vi "nn sendmsg.vi"(8 "error in (no error)":errorcluster, 9 "flags":i32, 10 "msghdr":T1, 11 "s":i32) -> (0 "error out":errorcluster, 3 "function return":i32)   [LabVIEW 2013, in "lvnano.lvlib"]
doc: "NN_EXPORT int nn_sendmsg (int s, const struct nn_msghdr *msghdr, int flags);"
uses:
  lvnano.lvlib
  get last error code.vi
  get error string from code.vi
  <vilib>/Utility/error.llb/Error Cluster From Error Code.vi
  lvnanomsg.dll
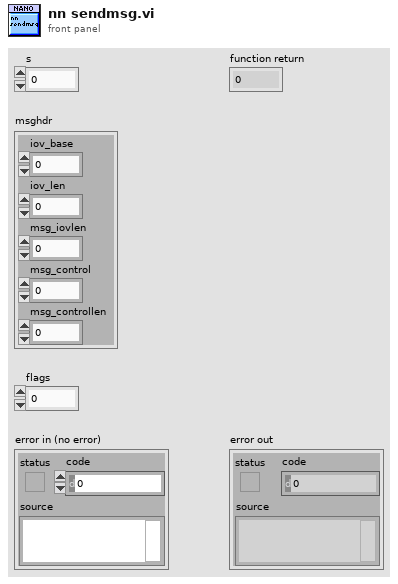
[diagram p1: front panel]
types:
  T1 = cluster{"iov_base":u32, "iov_len":u32, "msg_iovlen":i32, "msg_control":u32, "msg_controllen":u32}
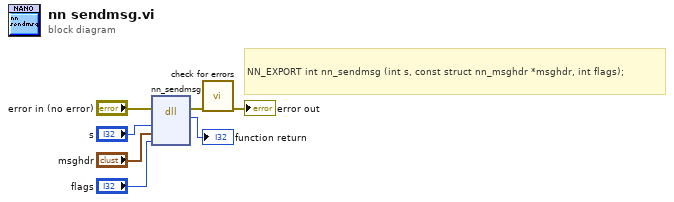
[diagram p0: block diagram]
diagram:
  # "NN_EXPORT int nn_sendmsg (int s, const struct nn_msghdr *msghdr, int flags);"
  n1 = dll-call lib="C:/Users/Daniel/Documents/nanomsg/lvnano/lvnanomsg.*" fn="nn_sendmsg"(error in="error in (no error)", "s"="s", "msghdr"="msghdr", "flags"="flags") -> (error out=w2:errorcluster, →"function return":i32)  [unwired: 5 in, 1 out]
  n2 = call "check for errors.vi"("error in"=w2) -> ("error out"=→"error out":errorcluster)  [unwired: 10 in]
